vi "Append New Element.vi"(8 "error in (no error)":errorcluster, 10 "New Element":refnum<class "xwpfDocument.Element.lvclass">, 11 "xwpfDocument in":refnum<class "xwpfDocument.lvclass">) -> (0 "error out":errorcluster, 3 "xwpfDocument out":refnum<class "xwpfDocument.lvclass">)   [LabVIEW 2017, in "Word_Specific.lvlib" / "xwpfDocument.lvclass"]
uses:
  xwpfDocument.lvclass
  xwpfDocument.Element/xwpfDocument.Element.lvclass
  xwpfDocument.lvclass/xwpfDocument.ctl
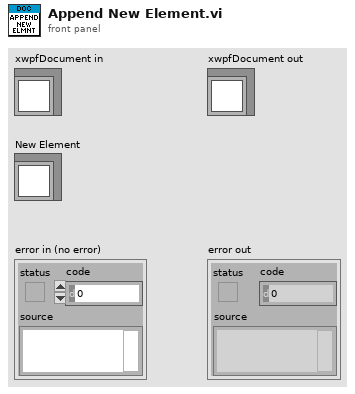
[diagram p1: front panel]
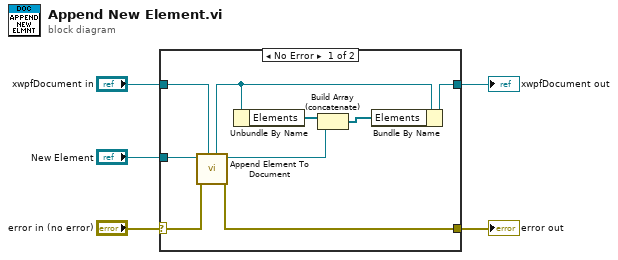
[diagram p0: block diagram]
diagram:
  n1 = case shown="No Error" "error in (no error)" {
    selector: "error in (no error)" -> [w13 w16]
    tunnel: [w11 w16] -> w4
    tunnel: [w9 w15] -> w2
    tunnel: "xwpfDocument in" -> [w12 w15]
    tunnel: "New Element" -> [w14 _]
    frame No Error {
      n2 = call "Append Element To Document.vi"("Document in"=w12, "error in (no error)"=w13, "xwpfDocument.Element in"=w14) -> ("error out"=w11:errorcluster, "xwpfDocument.Element out"=w6:refnum<class "xwpfDocument.Element.lvclass">, "Document out"=w10:refnum<class "xwpfDocument.lvclass">)  [unwired: 6 in]
      n3 = Unbundle By Name(w10) -> ("Elements"=w8:refnum<class "xwpfDocument.Element.lvclass">[])
      n4 = Build Array (concatenate)(w8, w6) -> (w7:refnum<class "xwpfDocument.Element.lvclass">[])
      n5 = Bundle By Name(cluster=w10, "Elements"=w7) -> (w9:refnum<class "xwpfDocument.lvclass">)
    }
    frame Error {
    }
  }
  "error out" <- w4
  "xwpfDocument out" <- w2
